vi "FilterInfoCoertion.vi"(1 "FilterInfo in":T1={"filter type"=enum."Lowpass", "high cutoff freq: fh"=0.45000000000000007, "low cutoff freq: fl"=0.12500000000000006, "order"=2} {"low cutoff freq: fl" format="%0.4f"; "high cutoff freq: fh" format="%0.2f"}) -> (0 "FilterInfo coerced":T1={"filter type"=enum."Lowpass", "high cutoff freq: fh"=0.45000000000000007, "low cutoff freq: fl"=0.12500000000000006, "order"=2} {"low cutoff freq: fl" format="%0.4f"; "high cutoff freq: fh" format="%0.2f"})   [LabVIEW 2016]
uses:
  FilterInfo.ctl
  <vilib>/Analysis/3filter.llb/Filter Passband Type.ctl
  <vilib>/Analysis/NI_AALBase.lvlib
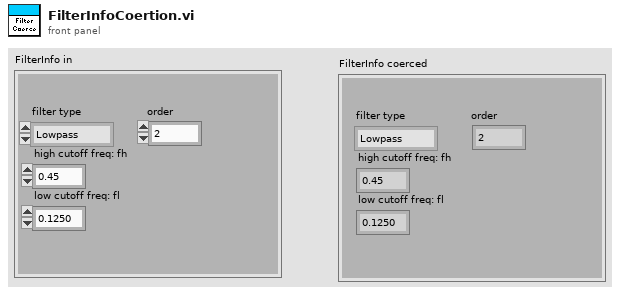
[diagram p1: front panel]
types:
  T1 = typedef "FilterInfo.ctl" = cluster{"filter type":T2, "high cutoff freq: fh":dbl, "low cutoff freq: fl":dbl, "order":i32}
  T2 = typedef "NI_AALBase.lvlib/Filter Passband Type.ctl" = enum32{"Lowpass", "Highpass", "Bandpass", "Bandstop"}
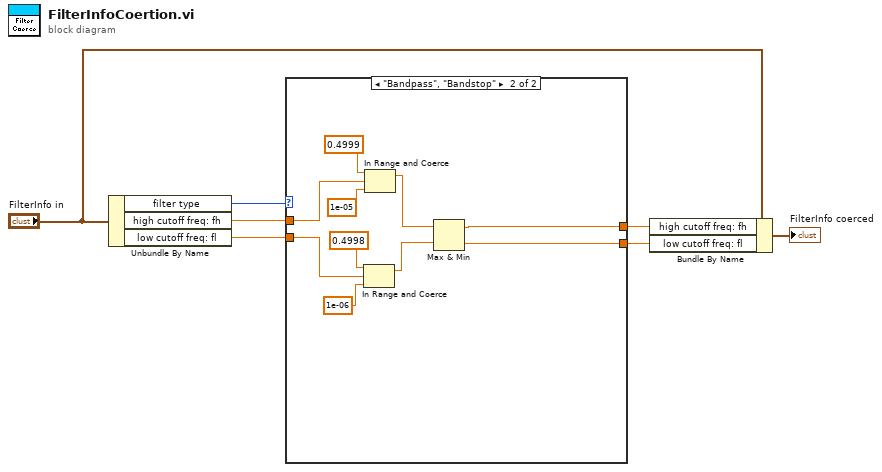
[diagram p0: block diagram]
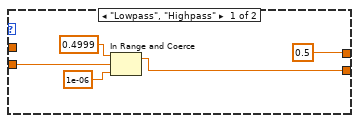
[diagram p2: hidden frame]
diagram:
  n1 = Unbundle By Name("FilterInfo in") -> ("filter type"=w7:T2, "high cutoff freq: fh"=w6:dbl, "low cutoff freq: fl"=w5:dbl)
  n2 = case shown="\"Bandpass\", \"Bandstop\"" w7 {
    tunnel: w6 -> [_ w17]
    tunnel: w5 -> [w12 w20]
    tunnel: [0.5 ("high cutoff freq: fh") w14] -> w3
    tunnel: [w9 w13] -> w2
    frame "Lowpass", "Highpass" {
      n3 = In Range and Coerce(upper limit=0.4999, x=w12, lower limit=1e-06) -> (coerced(x)=w9:dbl)  [unwired: 1 out]
    }
    frame "Bandpass", "Bandstop" {
      n4 = In Range and Coerce(upper limit=0.4998, x=w20, lower limit=1e-06) -> (coerced(x)=w15:dbl)  [unwired: 1 out]
      n5 = In Range and Coerce(upper limit=0.4999, x=w17, lower limit=1e-05) -> (coerced(x)=w16:dbl)  [unwired: 1 out]
      n6 = Max & Min(x=w16, y=w15) -> (max(x,y)=w14:dbl, min(x,y)=w13:dbl)
    }
  }
  n7 = Bundle By Name(cluster="FilterInfo in", "high cutoff freq: fh"=w3, "low cutoff freq: fl"=w2) -> (→"FilterInfo coerced":T1)
